vi "MTM2_getSample_axialActuatorAbsolutePositionSteps.vi"(8 "error in (no error)":errorcluster, 11 "axialActuatorAbsolutePositionSteps_Ctl":T1={"axialAbsolutePositionSteps[72]"=[0, 0, 0, 0, 0, 0, 0, 0, 0, 0, 0, 0, 0, 0, 0, 0, 0, 0, 0, 0, 0, 0, 0, 0, 0, 0, 0, 0, 0, 0, 0, 0, 0, 0, 0, 0, 0, 0, 0, 0, 0, 0, 0, 0, 0, 0, 0, 0, 0, 0, 0, 0, 0, 0, 0, 0, 0, 0, 0, 0, 0, 0, 0, 0, 0, 0, 0, 0, 0, 0, 0, 0]}) -> (0 "error out":errorcluster, 2 "function return":i32, 3 "axialActuatorAbsolutePositionSteps_Ctl out":T1)   [LabVIEW 2018, in "SALLV_MTM2.lvlib"]
doc: "int MTM2_shm_getSample_axialActuatorAbsolutePositionStepsLV(MTM2_axialActuatorAbsolutePositionStepsLV *axialActuatorAbsolutePositionSteps_Ctl );"
uses:
  SALLV_MTM2.lvlib
  DataTypes/axialActuatorAbsolutePositionSteps.ctl
  SALLV_MTM2.so
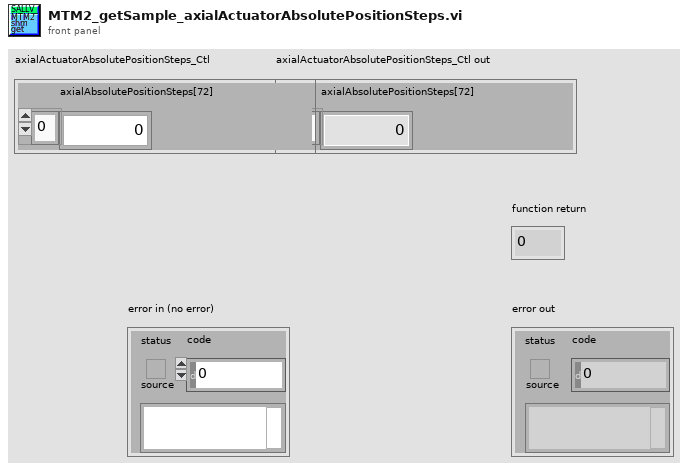
[diagram p1: front panel]
types:
  T1 = typedef "SALLV_MTM2.lvlib/axialActuatorAbsolutePositionSteps.ctl" = cluster{"axialAbsolutePositionSteps[72]":i32[]}
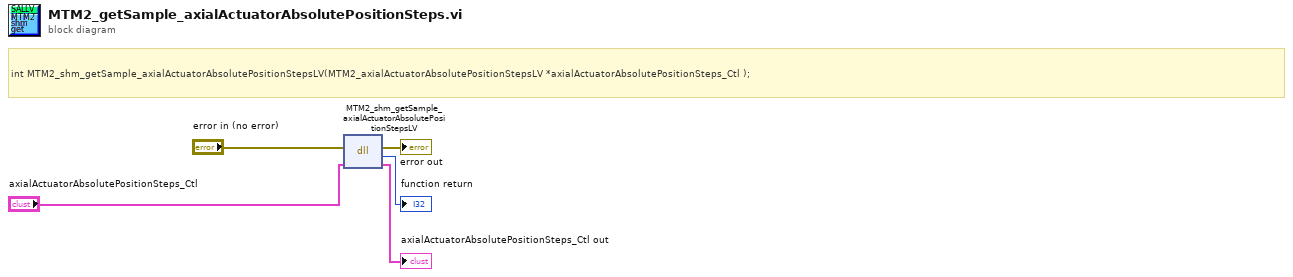
[diagram p0: block diagram]
diagram:
  # "int MTM2_shm_getSample_axialActuatorAbsolutePositionStepsLV(MTM2_axialActuatorAbsolutePositionStepsLV *axialActuatorAbsolutePositionSteps_Ctl );"
  n1 = dll-call lib="home/ttsai/Document/salApiMTM2/SALLV_MTM2/SALLV_MTM2.*" fn="MTM2_shm_getSample_axialActuatorAbsolutePositionStepsLV"(error in="error in (no error)", "axialActuatorAbsolutePositionSteps_Ctl"="axialActuatorAbsolutePositionSteps_Ctl") -> (error out=→"error out":errorcluster, →"function return":i32, "axialActuatorAbsolutePositionSteps_Ctl"=→"axialActuatorAbsolutePositionSteps_Ctl out":T1)  [unwired: 2 in, 1 out]
